vi "08T_LOGfilewrite.vi"(7 "refnum out":refnum<file>, 8 "Counters":T2, 9 "Flags":T1, 10 "Voltage":cluster{"Vin, V":dbl, "Vout, V":dbl} {"Vout, V" format="%#.2g"; "Vin, V" format="%#.5g"}, 11 "Temp":T3) -> ()   [LabVIEW 2017]
uses:
  <vilib>/Utility/error.llb/whitespace.ctl
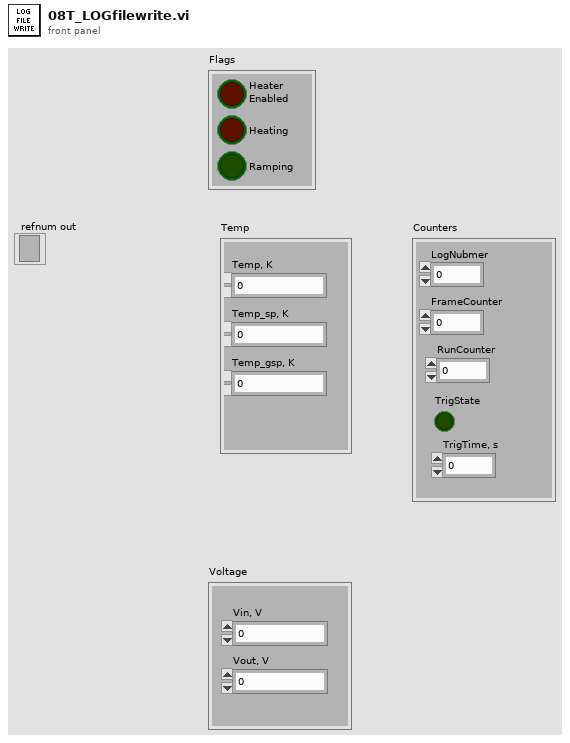
[diagram p1: front panel]
types:
  T1 = cluster{"Heater\nEnabled":bool, "Heating":bool, "Ramping":bool}
  T2 = cluster{"LogNubmer":i32, "FrameCounter":i32, "RunCounter":u32, "TrigState":bool, "TrigTime, s":dbl}
  T3 = cluster{"Temp_gsp, K":dbl, "Temp_sp, K":dbl, "Temp, K":dbl}
  T4 = typedef "whitespace.ctl" = u16
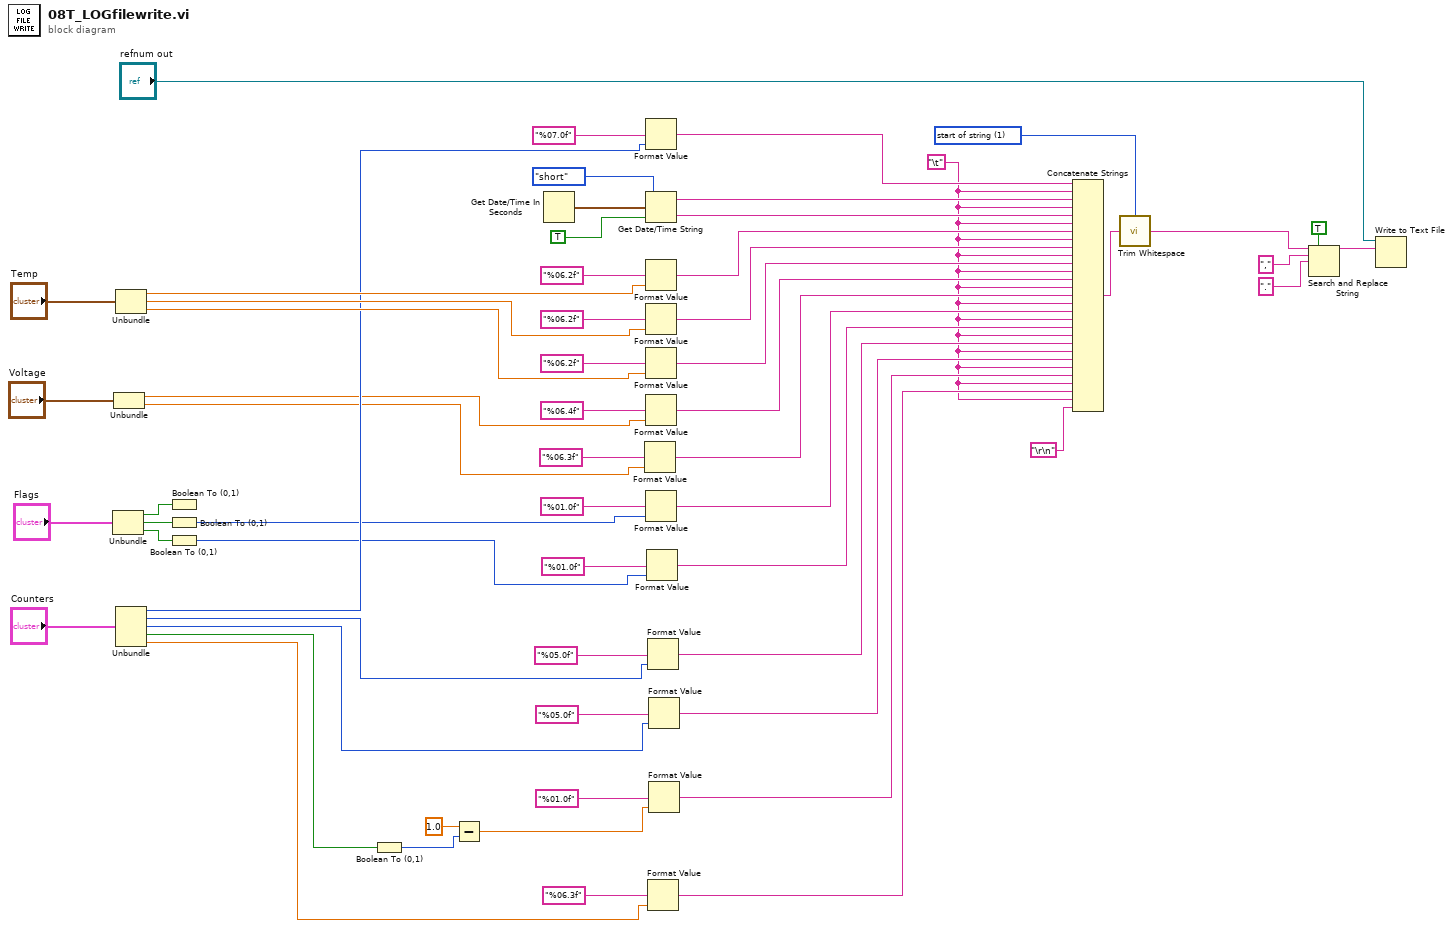
[diagram p0: block diagram]
diagram:
  w11 = "\t"
  w50 = T4 1 items=["both", "start of string", "end of string"] ("location (both)")
  n1 = Unbundle("Flags") -> ("Heater\nEnabled"=w6:bool, "Heating"=w5:bool, "Ramping"=w4:bool)
  n2 = Unbundle("Voltage") -> ("Vin, V"=w8:dbl, "Vout, V"=w7:dbl)
  n3 = Unbundle("Temp") -> ("Temp_gsp, K"=w36:dbl, "Temp_sp, K"=w35:dbl, "Temp, K"=w34:dbl)
  n4 = Unbundle("Counters") -> ("LogNubmer"=w29:i32, "FrameCounter"=w28:i32, "RunCounter"=w27:u32, "TrigState"=w13:bool, "TrigTime, s"=w15:dbl)
  n5 = Boolean To (0,1)(Boolean=w6) -> ()  [unwired: 1 out]
  n6 = Boolean To (0,1)(Boolean=w5) -> (0, 1=w2:i16)
  n7 = Boolean To (0,1)(Boolean=w4) -> (0, 1=w1:i16)
  n8 = Boolean To (0,1)(Boolean=w13) -> (0, 1=w14:i16)
  n9 = Subtract(x=1.0, y=w14) -> (x-y=w24:dbl)
  n10 = Get Date/Time In Seconds() -> (seconds since 1Jan1904=w57:timestamp)
  n11 = Format Value(format string="%06.3f", value (0)=w7) -> (output string=w17:string)  [unwired: 1 in]
  n12 = Format Value(format string="%07.0f", value (0)=w29) -> (output string=w47:string)  [unwired: 1 in]
  n13 = Get Date/Time String(date format (0)=enum16{"short", "long", "abbreviated"}."short", seconds (now)=w57, want seconds? (F)=TRUE) -> (date string=w48:string, time string=w49:string)
  n14 = Format Value(format string="%06.2f", value (0)=w36) -> (output string=w54:string)  [unwired: 1 in]
  n15 = Format Value(format string="%06.2f", value (0)=w35) -> (output string=w53:string)  [unwired: 1 in]
  n16 = Format Value(format string="%06.2f", value (0)=w34) -> (output string=w52:string)  [unwired: 1 in]
  n17 = Format Value(format string="%06.4f", value (0)=w8) -> (output string=w40:string)  [unwired: 1 in]
  n18 = Format Value(format string="%01.0f", value (0)=w2) -> (output string=w18:string)  [unwired: 1 in]
  n19 = Format Value(format string="%01.0f", value (0)=w1) -> (output string=w19:string)  [unwired: 1 in]
  n20 = Format Value(format string="%05.0f", value (0)=w28) -> (output string=w20:string)  [unwired: 1 in]
  n21 = Format Value(format string="%06.3f", value (0)=w15) -> (output string=w12:string)  [unwired: 1 in]
  n22 = Format Value(format string="%05.0f", value (0)=w27) -> (output string=w21:string)  [unwired: 1 in]
  n23 = Format Value(format string="%01.0f", value (0)=w24) -> (output string=w22:string)  [unwired: 1 in]
  n24 = Concatenate Strings(w47, w11, w48, w11, w49, w11, w54, w11, w53, w11, w52, w11, w40, w11, w17, w11, w18, w11, w19, w11, w20, w11, w21, w11, w22, w11, w12, w11, "\r\n") -> (w51:string)
  n25 = call <vilib>:"Trim Whitespace.vi"("string"=w51, "location (both)"=w50) -> ("trimmed string"=w43:string)
  n26 = Search and Replace String(replace all?=TRUE ("replace all? (F)"), input string=w43, search string=",", replace string="." ("replace string (\"\")")) -> (result string=w42:string)  [unwired: 4 in, 3 out]
  n27 = Write to Text File(file (use dialog)="refnum out", text=w42) -> ()  [unwired: 2 in, 3 out]
